vi "DIO_Ref_Num.vi"() -> (0 "DIO":T1)   [LabVIEW 2015]
uses:
  DIO_Type_Def.ctl
  <vilib>/Rock Robotics/WPI/Ultrasonic/WPI_SonarMB1010DigitalDeviceRef.ctl
  <vilib>/Rock Robotics/WPI/Counter/WPI_CounterDevRef.ctl
  <vilib>/Rock Robotics/SystemInterfaces/Counter/FPGA_CounterCtrSystemIndex.ctl
  <vilib>/Rock Robotics/WPI/Encoder/WPI_EncoderDevRef.ctl
  <vilib>/Rock Robotics/SystemInterfaces/Encoder/FPGA_EncoderIdx.ctl
  <vilib>/Rock Robotics/WPI/Encoder/WPI_EncoderType.ctl
  <vilib>/Rock Robotics/WPI/DigitalInput/WPI_DigitalInputDevRef.ctl
  <vilib>/Rock Robotics/SystemInterfaces/DIO/FPGA_DIOChannel.ctl
  <vilib>/Rock Robotics/WPI/Ultrasonic/WPI_SonarMB1010DigitalRefNum Registry Get.vi
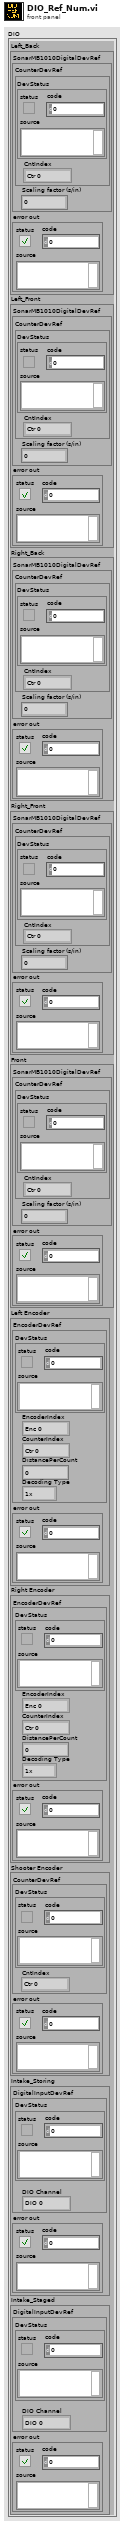
[diagram p1: front panel]
types:
  T1 = typedef "DIO_Type_Def.ctl" = cluster{"Left_Back":cluster{"SonarMB1010DigitalDevRef":T2, "error out":errorcluster}, "Left_Front":cluster{"SonarMB1010DigitalDevRef":T2, "error out":errorcluster}, "Right_Back":cluster{"SonarMB1010DigitalDevRef":T2, "error out":errorcluster}, "Right_Front":cluster{"SonarMB1010DigitalDevRef":T2, "error out":errorcluster}, "Front":cluster{"SonarMB1010DigitalDevRef":T2, "error out":errorcluster}, "Left Encoder":cluster{"EncoderDevRef":T5, "error out":errorcluster}, "Right Encoder":cluster{"EncoderDevRef":T5, "error out":errorcluster}, "Shooter Encoder":cluster{"CounterDevRef":T3, "error out":errorcluster}, "Intake_Storing":cluster{"DigitalInputDevRef":T8, "error out":errorcluster}, "Intake_Staged":cluster{"DigitalInputDevRef":T8, "error out":errorcluster}}
  T2 = typedef "WPI_SonarMB1010DigitalDeviceRef.ctl" = cluster{"CounterDevRef":T3, "Scaling factor (s/in)":dbl}
  T3 = typedef "WPI_CounterDevRef.ctl" = cluster{"DevStatus":errorcluster, "CntIndex":T4}
  T4 = typedef "FPGA_CounterCtrSystemIndex.ctl" = enum8{"Ctr 0", "Ctr 1", "Ctr 2", "Ctr 3", "Ctr 4", "Ctr 5", "Ctr 6", "Ctr 7", "Invalid"}
  T5 = typedef "WPI_EncoderDevRef.ctl" = cluster{"DevStatus":errorcluster, "EncoderIndex":T6, "CounterIndex":T4, "DistancePerCount":dbl, "Decoding Type":T7}
  T6 = typedef "FPGA_EncoderIdx.ctl" = enum8{"Enc 0", "Enc 1", "Enc 2", "Enc 3", "Enc 4", "Enc 5", "Enc 6", "Enc 7", "Invalid"}
  T7 = typedef "WPI_EncoderType.ctl" = enum16{"1x", "2x", "4x"}
  T8 = typedef "WPI_DigitalInputDevRef.ctl" = cluster{"DevStatus":errorcluster, "DIO Channel":T9}
  T9 = typedef "FPGA_DIOChannel.ctl" = enum8{"DIO 0", "DIO 1", "DIO 2", "DIO 3", "DIO 4", "DIO 5", "DIO 6", "DIO 7", "DIO 8", "DIO 9", "DIO MXP 0", "DIO MXP 1", "DIO MXP 2", "DIO MXP 3", "DIO MXP 4", "DIO MXP 5", "DIO MXP 6", "DIO MXP 7", "DIO MXP 8", "DIO MXP 9", "DIO MXP 10", "DIO MXP 11", "DIO MXP 12", "DIO MXP 13", "DIO MXP 14", "DIO MXP 15", "Invalid"}
  T10 = cluster{"CounterDevRef":T3, "error out":errorcluster}
  T11 = cluster{"DigitalInputDevRef":T8, "error out":errorcluster}
  T12 = cluster{"EncoderDevRef":T5, "error out":errorcluster}
  T13 = cluster{"SonarMB1010DigitalDevRef":T2, "error out":errorcluster}
  T14 = cluster{"Left_Back":cluster{"SonarMB1010DigitalDevRef":T2, "error out":errorcluster}, "Left_Front":cluster{"SonarMB1010DigitalDevRef":T2, "error out":errorcluster}, "Right_Back":cluster{"SonarMB1010DigitalDevRef":T2, "error out":errorcluster}, "Right_Front":cluster{"SonarMB1010DigitalDevRef":T2, "error out":errorcluster}, "Front":cluster{"SonarMB1010DigitalDevRef":T2, "error out":errorcluster}, "Left Encoder":cluster{"EncoderDevRef":T5, "error out":errorcluster}, "Right Encoder":cluster{"EncoderDevRef":T5, "error out":errorcluster}, "Shooter Encoder":cluster{"CounterDevRef":T3, "error out":errorcluster}, "Intake_Storing":cluster{"DigitalInputDevRef":T8, "error out":errorcluster}, "Intake_Staged":cluster{"DigitalInputDevRef":T8, "error out":errorcluster}}
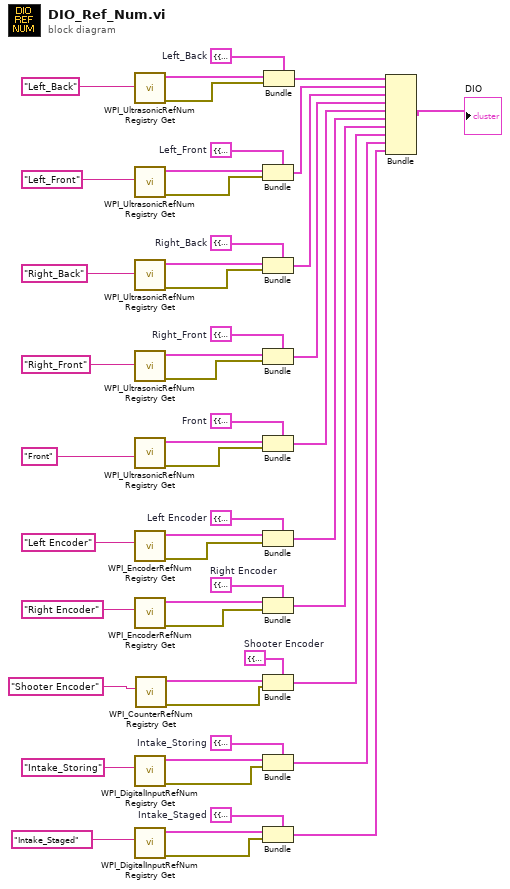
[diagram p0: block diagram]
diagram:
  w5 = T10 {"CounterDevRef"={"DevStatus"={"status"=FALSE, "code"=0, "source"=""}, "CntIndex"=enum."Ctr 0"}, "error out"={"status"=FALSE, "code"=0, "source"=""}}  # Shooter Encoder
  w39 = T11 {"DigitalInputDevRef"={"DevStatus"={"status"=FALSE, "code"=0, "source"=""}, "DIO Channel"=enum."DIO 0"}, "error out"={"status"=FALSE, "code"=0, "source"=""}}  # Intake_Staged
  w36 = T11 {"DigitalInputDevRef"={"DevStatus"={"status"=FALSE, "code"=0, "source"=""}, "DIO Channel"=enum."DIO 0"}, "error out"={"status"=FALSE, "code"=0, "source"=""}}  # Intake_Storing
  w30 = T12 {"EncoderDevRef"={"DevStatus"={"status"=FALSE, "code"=0, "source"=""}, "EncoderIndex"=enum."Enc 0", "CounterIndex"=enum."Ctr 0", "DistancePerCount"=0.0, "Decoding Type"=enum."1x"}, "error out"={"status"=FALSE, "code"=0, "source"=""}}  # Right Encoder
  w29 = T12 {"EncoderDevRef"={"DevStatus"={"status"=FALSE, "code"=0, "source"=""}, "EncoderIndex"=enum."Enc 0", "CounterIndex"=enum."Ctr 0", "DistancePerCount"=0.0, "Decoding Type"=enum."1x"}, "error out"={"status"=FALSE, "code"=0, "source"=""}}  # Left Encoder
  w24 = T13 {"SonarMB1010DigitalDevRef"={"CounterDevRef"={"DevStatus"={"status"=FALSE, "code"=0, "source"=""}, "CntIndex"=enum."Ctr 0"}, "Scaling factor (s/in)"=0.0}, "error out"={"status"=FALSE, "code"=0, "source"=""}}  # Front
  w19 = T13 {"SonarMB1010DigitalDevRef"={"CounterDevRef"={"DevStatus"={"status"=FALSE, "code"=0, "source"=""}, "CntIndex"=enum."Ctr 0"}, "Scaling factor (s/in)"=0.0}, "error out"={"status"=FALSE, "code"=0, "source"=""}}  # Right_Front
  w16 = T13 {"SonarMB1010DigitalDevRef"={"CounterDevRef"={"DevStatus"={"status"=FALSE, "code"=0, "source"=""}, "CntIndex"=enum."Ctr 0"}, "Scaling factor (s/in)"=0.0}, "error out"={"status"=FALSE, "code"=0, "source"=""}}  # Right_Back
  w11 = T13 {"SonarMB1010DigitalDevRef"={"CounterDevRef"={"DevStatus"={"status"=FALSE, "code"=0, "source"=""}, "CntIndex"=enum."Ctr 0"}, "Scaling factor (s/in)"=0.0}, "error out"={"status"=FALSE, "code"=0, "source"=""}}  # Left_Front
  w8 = T13 {"SonarMB1010DigitalDevRef"={"CounterDevRef"={"DevStatus"={"status"=FALSE, "code"=0, "source"=""}, "CntIndex"=enum."Ctr 0"}, "Scaling factor (s/in)"=0.0}, "error out"={"status"=FALSE, "code"=0, "source"=""}}  # Left_Back
  n1 = call-poly <vilib>:"WPI_UltrasonicRefNum Registry Get.vi"("refnum name"="Left_Back") -> ("error out"=w7:errorcluster, "SonarMB1010DigitalDevRef"=w6:T2)  [unwired: 9 in]
  n2 = call-poly <vilib>:"WPI_UltrasonicRefNum Registry Get.vi"("refnum name"="Left_Front") -> ("error out"=w12:errorcluster, "SonarMB1010DigitalDevRef"=w13:T2)  [unwired: 9 in]
  n3 = call-poly <vilib>:"WPI_UltrasonicRefNum Registry Get.vi"("refnum name"="Right_Back") -> ("error out"=w15:errorcluster, "SonarMB1010DigitalDevRef"=w14:T2)  [unwired: 9 in]
  n4 = call-poly <vilib>:"WPI_UltrasonicRefNum Registry Get.vi"("refnum name"="Right_Front") -> ("error out"=w20:errorcluster, "SonarMB1010DigitalDevRef"=w21:T2)  [unwired: 9 in]
  n5 = call-poly <vilib>:"WPI_UltrasonicRefNum Registry Get.vi"("refnum name"="Front") -> ("error out"=w23:errorcluster, "SonarMB1010DigitalDevRef"=w22:T2)  [unwired: 9 in]
  n6 = call <vilib>:"WPI_EncoderRefNum Registry Get.vi"("refnum name"="Left Encoder") -> ("error out"=w27:errorcluster, "EncoderDevRef"=w26:T5)  [unwired: 9 in]
  n7 = call <vilib>:"WPI_EncoderRefNum Registry Get.vi"("refnum name"="Right Encoder") -> ("error out"=w32:errorcluster, "EncoderDevRef"=w33:T5)  [unwired: 9 in]
  n8 = call <vilib>:"WPI_DigitalInputRefNum Registry Get.vi"("refnum name"="Intake_Storing") -> ("error out"=w35:errorcluster, "DigitalInputDevRef"=w34:T8)  [unwired: 9 in]
  n9 = call <vilib>:"WPI_DigitalInputRefNum Registry Get.vi"("refnum name"="Intake_Staged") -> ("error out"=w40:errorcluster, "DigitalInputDevRef"=w41:T8)  [unwired: 9 in]
  n10 = call <vilib>:"WPI_CounterRefNum Registry Get.vi"("refnum name"="Shooter Encoder") -> ("error out"=w3:errorcluster, "CounterDevRef"=w4:T3)  [unwired: 9 in]
  n11 = Bundle(cluster=w11, "SonarMB1010DigitalDevRef"=w13, "error out"=w12) -> (w43:T13)
  n12 = Bundle(cluster=w16, "SonarMB1010DigitalDevRef"=w14, "error out"=w15) -> (w44:T13)
  n13 = Bundle(cluster=w19, "SonarMB1010DigitalDevRef"=w21, "error out"=w20) -> (w45:T13)
  n14 = Bundle(cluster=w24, "SonarMB1010DigitalDevRef"=w22, "error out"=w23) -> (w46:T13)
  n15 = Bundle(cluster=w29, "EncoderDevRef"=w26, "error out"=w27) -> (w47:T12)
  n16 = Bundle(cluster=w30, "EncoderDevRef"=w33, "error out"=w32) -> (w48:T12)
  n17 = Bundle(cluster=w5, "CounterDevRef"=w4, "error out"=w3) -> (w49:T10)
  n18 = Bundle(cluster=w36, "DigitalInputDevRef"=w34, "error out"=w35) -> (w50:T11)
  n19 = Bundle(cluster=w39, "DigitalInputDevRef"=w41, "error out"=w40) -> (w51:T11)
  n20 = Bundle(cluster=w8, "SonarMB1010DigitalDevRef"=w6, "error out"=w7) -> (w42:T13)
  n21 = Bundle("Left_Back"=w42, "Left_Front"=w43, "Right_Back"=w44, "Right_Front"=w45, "Front"=w46, "Left Encoder"=w47, "Right Encoder"=w48, "Shooter Encoder"=w49, "Intake_Storing"=w50, "Intake_Staged"=w51) -> (→"DIO":T14)  [unwired: 1 in]
